vi "Main.vi"() -> ()   [LabVIEW 2013]
panel:
  in  "Tab Control":T1(tab)
  in  "General Information Clust":T2 {"Date" format="%<%H:%M\n%x>T"}
  out "B Reverse":bool
  out "B Forward":bool
  out "A Reverse":bool
  out "A Forward":bool
  in  "B Side XDCR":dbl format="%_6g"
  in  "A Side XDCR":dbl format="%_6g"
  in  "Record Pres.":bool
  out "Manifold Leak Test Graph":dbl[](graph)
  in  "Close Valves":bool
  out "Pressure Test Graph":dbl[](graph)
  in  "Finished":bool
  in  "Start Recored Pressure Verification":bool
  in  "Finished Flow Mode":bool
  in  "Start Flow Verification":bool
  out "Flow Verification":dbl[](graph)
  in  "Finish 2":bool
  in  "Cancel":bool
  in  "Finish":bool
  in  "Back":bool
  in  "Next":bool
  # "VPA Quality Control Checklist"
  # "Assembly Checklist"
  # "Transducer and Limit Switch Tests"
  # "Ensure voltage of transducers are calibrated so they do not give negative numbers. Voltage can be adjusted by taking off the screw that is \nlabeled \"Zero\" and turning the screw. Value needs to be less than .05 but greater than 0."
  # "Verify limit switch boards work by blacing a flag inplace of interruptors."
  # "Check Pump Function"
  # "Initialize pump and run in flow mode at 10% max speed for several minutes. Verify pump is operating normally (cylinders are stroking proper length, they do not run up too far when matching pressure, there is no air in the lines, etc.)"
  # "Manifold/Cylinder Leak Test"
  # "1. In pressure control mode, ramp to 95% max pressure."
  # "2. Close all manifold valves"
  # "3. Stop pressure control"
  # "4. Open External Valve. Record the pressure in the table below for 10 minutes."
  # "5. Start recording the pressure."
  # "Calibrate Pressure Transducers"
  # "Pressure Mode Verification"
  # "1. Close the external valve and ramp to 95% max pressure."
  # "2. Start recording pressure."
  # "3. Crack the external valve and allow valves to transition twice."
  # "Flow Mode Verification"
  # "1. Flow at max flow rate for 10 minutes."
  # "2. Run at max flow rate with 95% backpressure and record data for 2 minutes."
  # "Manifold/Cylinder Leak Test"
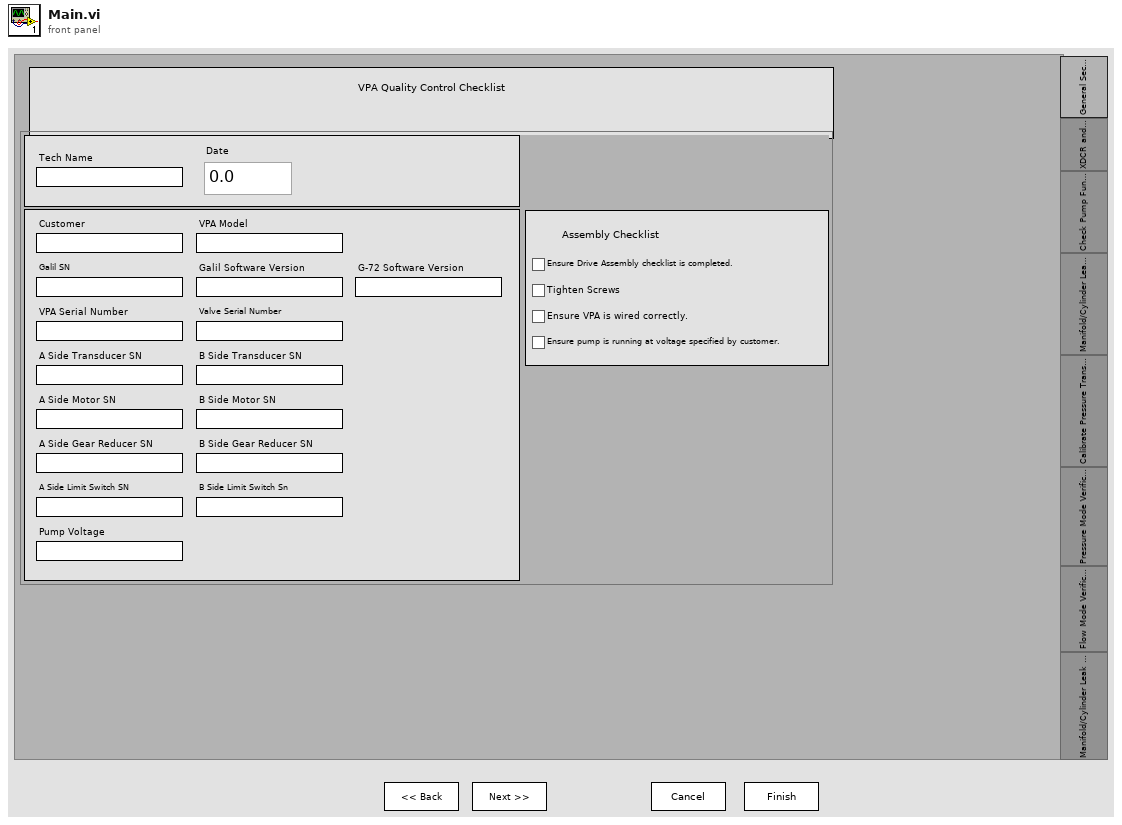
[diagram p1: front panel]
types:
  T1 = enum32{"General Section", "XDCR and LS", "Check Pump Function", "Manifold/Cylinder Leak Test", "Calibrate Pressure Transducers", "Pressure Mode Verification", "Flow Mode Verification", "Manifold/Cylinder Leak Test 5"}
  T2 = cluster{"Tech Name":string, "Customer":string, "Date":dbl, "VPA Model":string, "VPA Serial Number":string, "A Side Transducer SN":string, "B Side Transducer SN":string, "Valve Serial Number":string, "Galil SN":string, "Galil Software Version":string, "A Side Gear Reducer SN":string, "B Side Gear Reducer SN":string, "A Side Motor SN":string, "B Side Motor SN":string, "G-72 Software Version":string, "A Side Limit Switch SN":string, "B Side Limit Switch Sn":string, "Pump Voltage":string, "Ensure Drive Assembly checklist is completed.":bool, "Tighten Screws":bool, "Ensure VPA is wired correctly.":bool, "Ensure pump is running at voltage specified by customer.":bool}
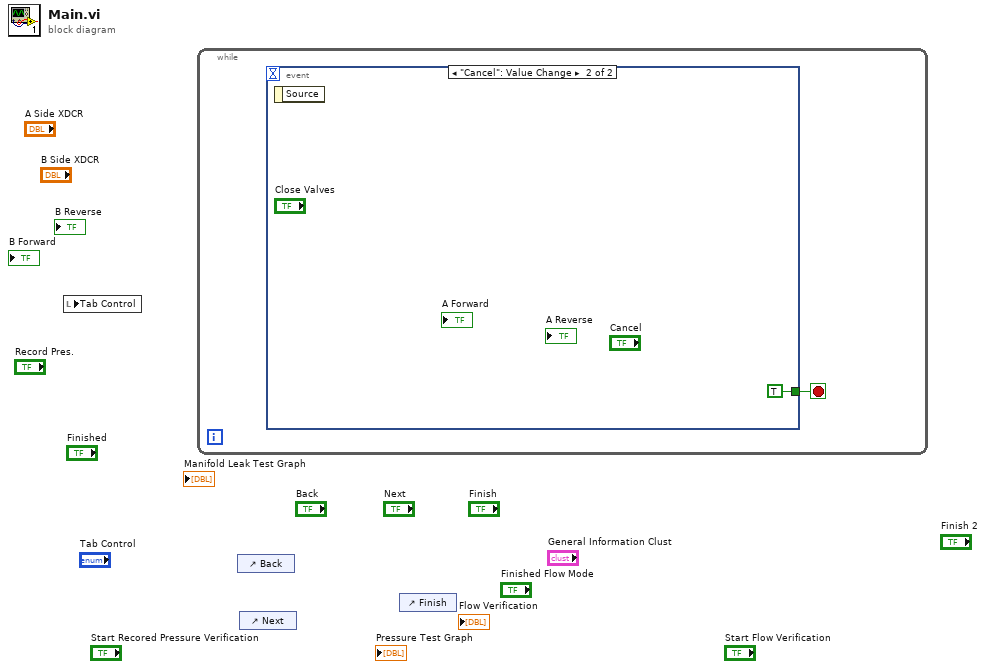
[diagram p0: block diagram]
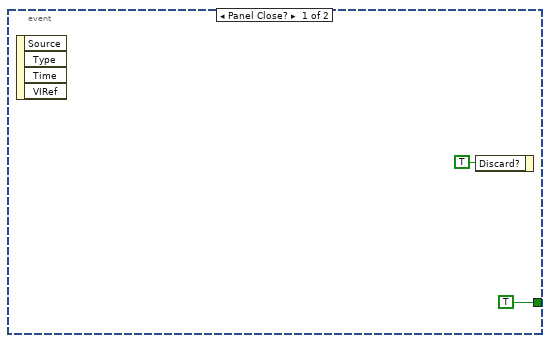
[diagram p2: hidden frame]
diagram:
  n1 = local read "Tab Control"() -> ()  [unwired: 1 in]
  n2 = while {
    stop <- w1 stop-if-true
    n3 = event shown="[1] \"Cancel\": Value Change" {
      selector: _ -> [_ _]
      dyn-events: _ -> [_ _]
      timeout: _ -> [_ _]
      tunnel: [TRUE TRUE] -> w1
      event Panel Close? {
        n4 = event-data() -> ()  [unwired: 1 in, 4 out]
        n5 = event-data("Discard?"=TRUE) -> ()  [unwired: 1 in, 1 out]
      }
      event "Cancel": Value Change {
        n6 = event-data() -> ()  [unwired: 1 in, 1 out]
      }
    }
  }
  n7 = control-ref of="Back"() -> ()  [unwired: 1 out]
  n8 = control-ref of="Next"() -> ()  [unwired: 1 out]
  n9 = control-ref of="Finish"() -> ()  [unwired: 1 out]
